vi "Fetch Real Time Eye Measurements.vi"(8 "error in (no error)":errorcluster, 11 "VISA resource name":refnum<visa-resource-name>) -> (0 "error out":errorcluster, 1 "Eye Width":dbl, 2 "Eye Height":dbl, 3 "VISA resource name out":refnum<visa-resource-name>, 5 "UI Intervals Folded Into Real-Time Eye":i32)   [LabVIEW 2015, in "Agilent 2000 3000 X-Series.lvlib"]
doc: "Fetches measurements from real-time eye analysis.\n\n<b>Note:</b>\nThis VI is specific to the 6000-X Series oscilloscopes. These features are not available on other models."
uses:
  <instrlib>/Agilent 2000 3000 X-Series/Agilent 2000 3000 X-Series.lvlib
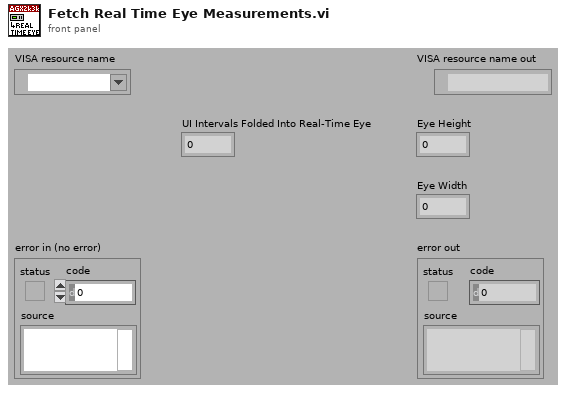
[diagram p1: front panel]
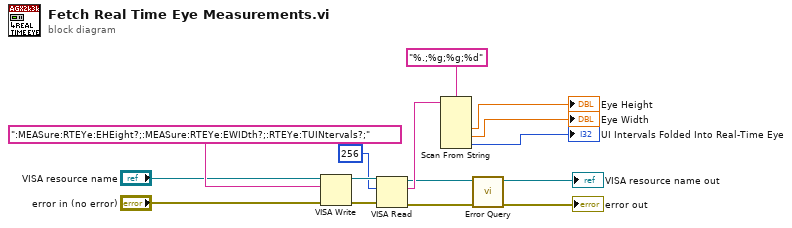
[diagram p0: block diagram]
diagram:
  n1 = VISA Write(VISA resource name="VISA resource name", write buffer=":MEASure:RTEYe:EHEight?;:MEASure:RTEYe:EWIDth?;:RTEYe:TUINtervals?;", error in (no error)="error in (no error)") -> (VISA resource name out=w11:refnum<visa-resource-name>, error out=w12:errorcluster)  [unwired: 1 out]
  n2 = VISA Read(VISA resource name=w11, byte count=u32 256, error in (no error)=w12) -> (VISA resource name out=w4:refnum<visa-resource-name>, read buffer=w9:string, error out=w3:errorcluster)  [unwired: 1 out]
  n3 = Scan From String(format string="%.;%g;%g;%d", input string=w9) -> (output 1=→"Eye Height":dbl, output 2=→"Eye Width":dbl, output 3=→"UI Intervals Folded Into Real-Time Eye":i32)  [unwired: 5 in, 3 out]
  n4 = call <instrlib>:"Error Query.vi"("error in (no error)"=w3, "VISA resource name"=w4) -> ("error out"=→"error out":errorcluster, "VISA resource name out"=→"VISA resource name out":refnum<visa-resource-name>)  [unwired: 6 in, 2 out]
